vi "Two Fgen Module.vi"() -> ()   [LabVIEW 2021]
panel:
  in  "I3C Generator Fgen Channel":string
  in  "I3C waveform":T1(ring)=enum."Noise"
  in  "I3C frequency":dbl=6.0
  in  "I3C amplitude":dbl=6.0
  in  "I3C Generator Fgen":refnum<k15>
  out "I3C Duration":dbl
  in  "duration":dbl
  out "I2C Duration":dbl
  in  "I2C Generator Fgen":refnum<k15>
  in  "I2C amplitude":dbl=6.0
  in  "I2C frequency":dbl=6.0
  in  "I2C waveform":T1(ring)=enum."Noise"
  in  "I2C Generator Fgen Channel":string
  out "error out":errorcluster
  in  "error in":errorcluster
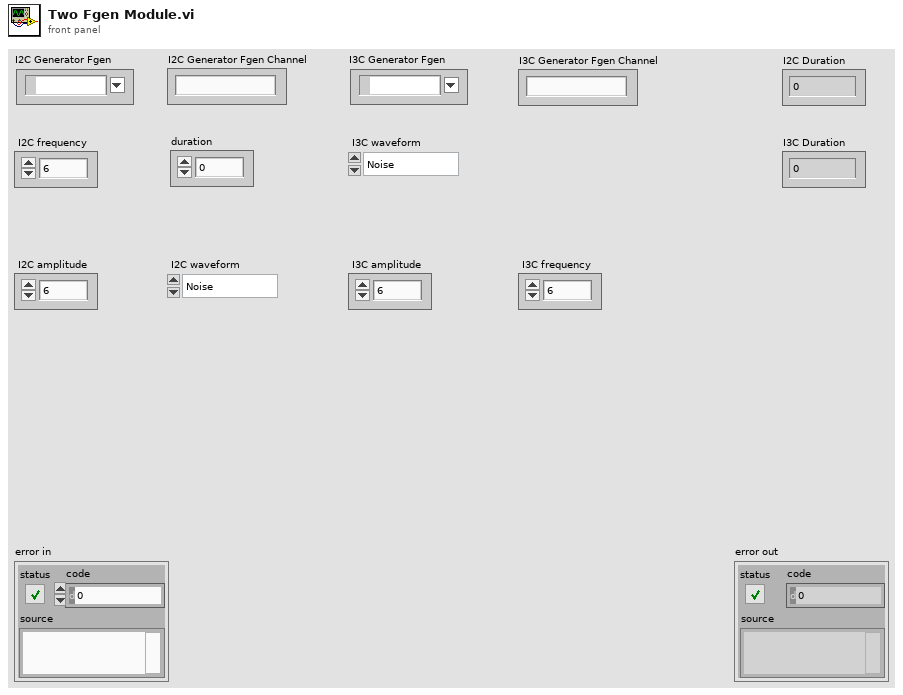
[diagram p1: front panel]
types:
  T1 = enum32{"Sine", "Square", "Triangle", "Ramp Up", "Ramp Down", "DC", "Noise", "User"}
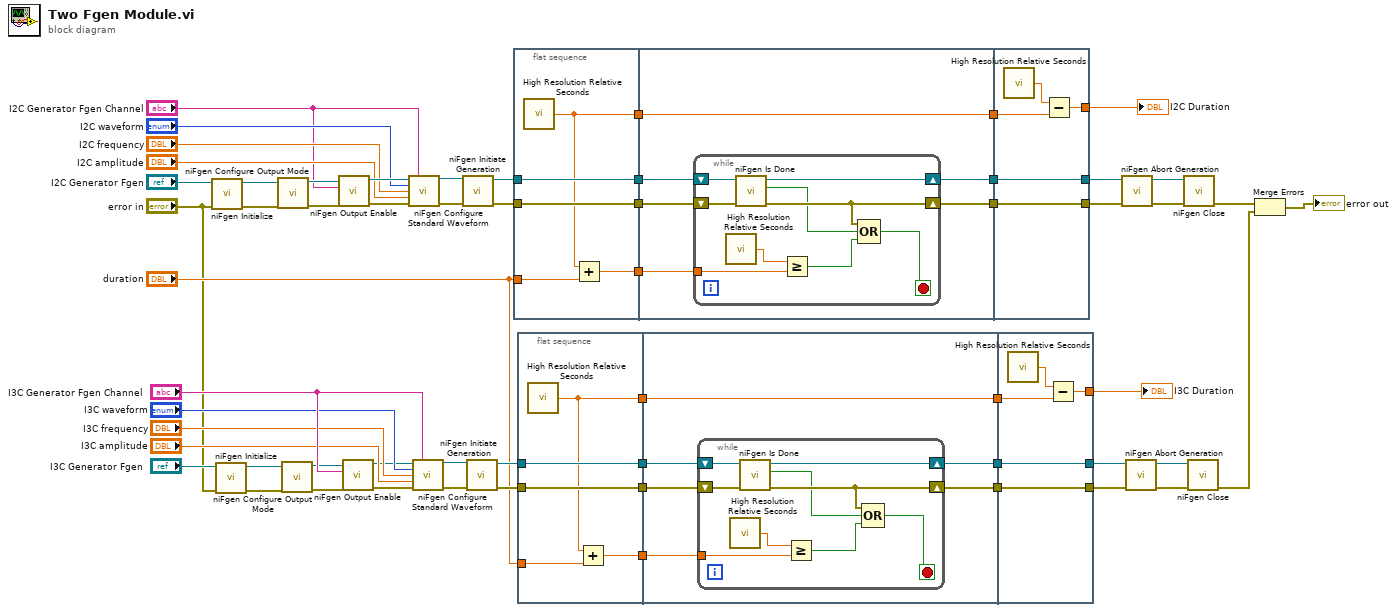
[diagram p0: block diagram]
diagram:
  n1 = call <instrlib>:"niFgen Initialize.vi"("error in (no error)"="error in", "Resource Name"="I2C Generator Fgen") -> ("error out"=w56:errorcluster, "Instrument Handle Out"=w59:refnum<k15>)  [unwired: 8 in]
  n2 = call <instrlib>:"niFgen Initialize.vi"("error in (no error)"="error in", "Resource Name"="I3C Generator Fgen") -> ("error out"=w8:errorcluster, "Instrument Handle Out"=w5:refnum<k15>)  [unwired: 8 in]
  n3 = call <instrlib>:"niFgen Configure Output Mode.vi"("error in (no error)"=w56, "Instrument Handle"=w59) -> ("error out"=w45:errorcluster, "Instrument Handle Out"=w55:refnum<k15>)  [unwired: 7 in]
  n4 = call <instrlib>:"niFgen Configure Output Mode.vi"("error in (no error)"=w8, "Instrument Handle"=w5) -> ("error out"=w18:errorcluster, "Instrument Handle Out"=w9:refnum<k15>)  [unwired: 7 in]
  n5 = call <instrlib>:"niFgen Output Enable.vi"("error in (no error)"=w45, "Channel Name"="I2C Generator Fgen Channel", "Instrument Handle"=w55) -> ("error out"=w57:errorcluster, "Instrument Handle Out"=w54:refnum<k15>)  [unwired: 7 in]
  n6 = call <instrlib>:"niFgen Output Enable.vi"("error in (no error)"=w18, "Channel Name"="I3C Generator Fgen Channel", "Instrument Handle"=w9) -> ("error out"=w7:errorcluster, "Instrument Handle Out"=w10:refnum<k15>)  [unwired: 7 in]
  n7 = call <instrlib>:"niFgen Configure Standard Waveform.vi"("Instrument Handle"=w54, "Channel Name"="I2C Generator Fgen Channel", "Waveform"="I2C waveform", "Frequency"="I2C frequency", "Amplitude"="I2C amplitude", "error in (no error)"=w57) -> ("Instrument Handle Out"=w53:refnum<k15>, "error out"=w58:errorcluster)  [unwired: 8 in]
  n8 = call <instrlib>:"niFgen Configure Standard Waveform.vi"("Instrument Handle"=w10, "Channel Name"="I3C Generator Fgen Channel", "Waveform"="I3C waveform", "Frequency"="I3C frequency", "Amplitude"="I3C amplitude", "error in (no error)"=w7) -> ("Instrument Handle Out"=w11:refnum<k15>, "error out"=w6:errorcluster)  [unwired: 8 in]
  n9 = call <instrlib>:"niFgen Initiate Generation.vi"("error in (no error)"=w58, "Instrument Handle"=w53) -> ("error out"=w50:errorcluster, "Instrument Handle Out"=w52:refnum<k15>)  [unwired: 8 in]
  n10 = call <instrlib>:"niFgen Initiate Generation.vi"("error in (no error)"=w6, "Instrument Handle"=w11) -> ("error out"=w14:errorcluster, "Instrument Handle Out"=w12:refnum<k15>)  [unwired: 8 in]
  n11 = flat-sequence {
    tunnel: w50 -> [w63]
    tunnel: w52 -> [w64]
    tunnel: [w64] -> w39
    tunnel: [w63] -> w38
    tunnel: [w62] -> w34
    tunnel: "duration" -> [w61]
    tunnel: [w60] -> w32
    tunnel: w39 -> [w70]
    tunnel: w38 -> [w68]
    tunnel: [w69] -> w37
    tunnel: [w67] -> w36
    tunnel: [w66] -> w35
    tunnel: w34 -> [w66]
    tunnel: w32 -> [w65]
    tunnel: [w83] -> w49
    tunnel: [w84] -> w51
    tunnel: w37 -> [w84]
    tunnel: w36 -> [w83]
    tunnel: w35 -> [w81]
    tunnel: [w80] -> w33
    frame #0 {
      n12 = call <vilib>:"High Resolution Relative Seconds.vi"() -> ("relative seconds"=w62:dbl)
      n13 = Add(x=w62, y=w61) -> (x+y=w60:dbl)
    }
    frame #1 {
      n14 = while {
        shift-right: [w78] -> w69
        shift-left: w70 -> [w79]
        shift-right: [w76] -> w67
        shift-left: w68 -> [w77]
        tunnel: w65 -> [w73]
        stop <- w75 stop-if-true
        n15 = call <vilib>:"High Resolution Relative Seconds.vi"() -> ("relative seconds"=w74:dbl)
        n16 = call <instrlib>:"niFgen Is Done.vi"("error in (no error)"=w77, "Instrument Handle"=w79) -> ("error out"=w76:errorcluster, "Done"=w71:bool, "Instrument Handle Out"=w78:refnum<k15>)  [unwired: 7 in]
        n17 = Greater Or Equal?(x=w74, y=w73) -> (x >= y?=w72:bool)
        n18 = Compound Arithmetic op=OR(w76, w71, w72) -> (w75:bool)
      }
    }
    frame #2 {
      n19 = call <vilib>:"High Resolution Relative Seconds.vi"() -> ("relative seconds"=w82:dbl)
      n20 = Subtract(x=w82, y=w81) -> (x-y=w80:dbl)
    }
  }
  n21 = flat-sequence {
    tunnel: w14 -> [w88]
    tunnel: w12 -> [w89]
    tunnel: [w89] -> w31
    tunnel: [w88] -> w30
    tunnel: [w87] -> w29
    tunnel: "duration" -> [w86]
    tunnel: [w85] -> w28
    tunnel: w31 -> [w95]
    tunnel: w30 -> [w93]
    tunnel: [w94] -> w27
    tunnel: [w92] -> w26
    tunnel: [w91] -> w25
    tunnel: w29 -> [w91]
    tunnel: w28 -> [w90]
    tunnel: [w108] -> w15
    tunnel: [w109] -> w13
    tunnel: w27 -> [w109]
    tunnel: w26 -> [w108]
    tunnel: w25 -> [w106]
    tunnel: [w105] -> w24
    frame #0 {
      n22 = call <vilib>:"High Resolution Relative Seconds.vi"() -> ("relative seconds"=w87:dbl)
      n23 = Add(x=w87, y=w86) -> (x+y=w85:dbl)
    }
    frame #1 {
      n24 = while {
        shift-right: [w103] -> w94
        shift-left: w95 -> [w104]
        shift-right: [w101] -> w92
        shift-left: w93 -> [w102]
        tunnel: w90 -> [w98]
        stop <- w100 stop-if-true
        n25 = call <vilib>:"High Resolution Relative Seconds.vi"() -> ("relative seconds"=w99:dbl)
        n26 = call <instrlib>:"niFgen Is Done.vi"("error in (no error)"=w102, "Instrument Handle"=w104) -> ("error out"=w101:errorcluster, "Done"=w96:bool, "Instrument Handle Out"=w103:refnum<k15>)  [unwired: 7 in]
        n27 = Greater Or Equal?(x=w99, y=w98) -> (x >= y?=w97:bool)
        n28 = Compound Arithmetic op=OR(w101, w96, w97) -> (w100:bool)
      }
    }
    frame #2 {
      n29 = call <vilib>:"High Resolution Relative Seconds.vi"() -> ("relative seconds"=w107:dbl)
      n30 = Subtract(x=w107, y=w106) -> (x-y=w105:dbl)
    }
  }
  n31 = call <instrlib>:"niFgen Abort Generation.vi"("error in (no error)"=w49, "Instrument Handle"=w51) -> ("error out"=w47:errorcluster, "Instrument Handle Out"=w48:refnum<k15>)  [unwired: 8 in]
  n32 = call <instrlib>:"niFgen Abort Generation.vi"("error in (no error)"=w15, "Instrument Handle"=w13) -> ("error out"=w17:errorcluster, "Instrument Handle Out"=w16:refnum<k15>)  [unwired: 8 in]
  n33 = call <instrlib>:"niFgen Close.vi"("error in (no error)"=w47, "Instrument Handle"=w48) -> ("error out"=w46:errorcluster)  [unwired: 9 in]
  n34 = call <instrlib>:"niFgen Close.vi"("error in (no error)"=w17, "Instrument Handle"=w16) -> ("error out"=w2:errorcluster)  [unwired: 9 in]
  n35 = Merge Errors(w46, w2) -> (→"error out":errorcluster)
  "I2C Duration" <- w33
  "I3C Duration" <- w24
